vi "Timer.vi"() -> ()   [LabVIEW 2015]
panel:
  in  "Numeric":dbl
  out "Meter":dbl(knob) scale=0.0..60.0
  in  "stop":bool
  out "Time":dbl
  out "Gauge":dbl(knob) scale=0.0..60.0
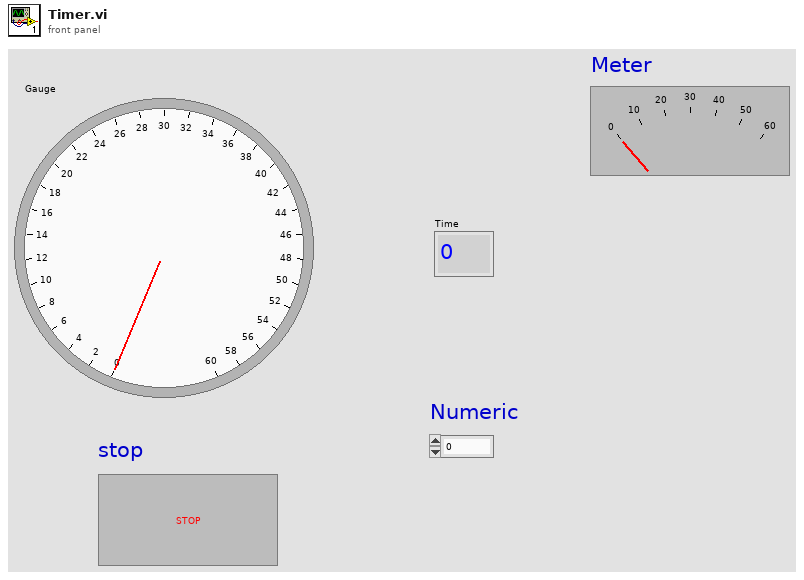
[diagram p1: front panel]
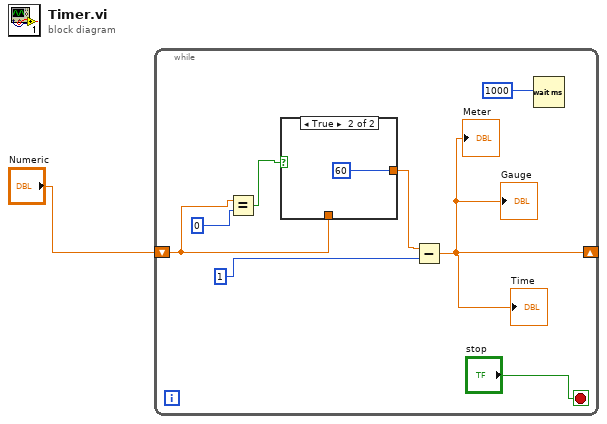
[diagram p0: block diagram]
diagram:
  n1 = while {
    shift-right: [w2] -> _
    shift-left: "Numeric" -> [w4]
    stop <- "stop" stop-if-true
    n2 = Equal?(x=w4, y=0) -> (x = y?=w6:bool)
    n3 = case shown="True" w6 {
      tunnel: [w10 60] -> w5
      tunnel: w4 -> [w10 _]
      frame False {
      }
      frame True {
      }
    }
    n4 = Subtract(x=w5, y=1) -> (x-y=w2:dbl)
    "Gauge" <- w2
    "Time" <- w2
    "Meter" <- w2
    n5 = Wait (ms)(milliseconds to wait=1000) -> ()  [unwired: 1 out]
  }
